vi "Bi Directional Trajectory.vi"(4 "Return Time":dbl, 6 "Go Time":dbl, 7 "Traj Start":i32(knob) scale=0.0..2.0, 10 "Trajectory Settings":cluster{"Total Time":dbl, "Control Freq":dbl}) -> (1 "Return Next Time":dbl, 2 "Go Next Time":dbl, 3 "Phase":dbl)   [LabVIEW 2021]
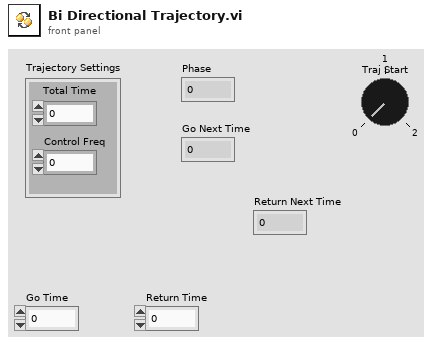
[diagram p1: front panel]
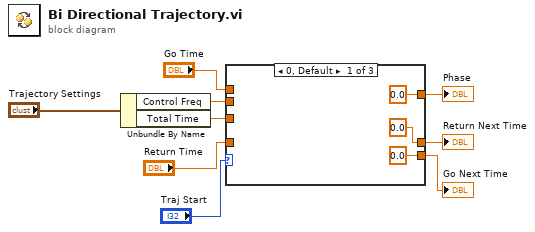
[diagram p0: block diagram]
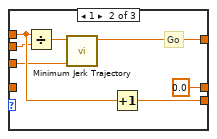
[diagram p2: hidden frame]
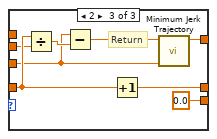
[diagram p3: hidden frame]
diagram:
  n1 = Unbundle By Name("Trajectory Settings") -> ("Control Freq"=w1:dbl, "Total Time"=w2:dbl)
  n2 = case shown="0, Default" "Traj Start" {
    tunnel: "Go Time" -> [_ w17 _]
    tunnel: [0.0 w19 0.0] -> w6
    tunnel: [0.0 ("ref_x (mm)") w16 w27] -> w7
    tunnel: "Return Time" -> [_ _ w25]
    tunnel: [0.0 0.0 w20] -> w9
    tunnel: w2 -> [_ w14 w22]
    tunnel: w1 -> [_ w13 w21]
    frame 0, Default {
    }
    frame 1 {
      # "Go"
      n3 = Divide(x=w17, y=w13) -> (x/y=w18:dbl)
      n4 = call "Minimum Jerk Trajectory.vi"("total time"=w14, "t (sec)"=w18) -> ("ref_x (mm)"=w16:dbl)  [unwired: 8 in, 1 out]
      n5 = Increment(x=w17) -> (x+1=w19:dbl)
    }
    frame 2 {
      # "Return"
      n6 = Divide(x=w25, y=w21) -> (x/y=w24:dbl)
      n7 = Subtract(x=w22, y=w24) -> (x-y=w23:dbl)
      n8 = Increment(x=w25) -> (x+1=w20:dbl)
      n9 = call "Minimum Jerk Trajectory.vi"("total time"=w22, "t (sec)"=w23) -> ("ref_x (mm)"=w27:dbl)  [unwired: 8 in, 1 out]
    }
  }
  "Return Next Time" <- w9
  "Phase" <- w7
  "Go Next Time" <- w6
